vi "PH_ForceSensor.read DB.vi"(1 "Force Sensor Instance":string, 5 "error in (no error)":errorcluster) -> (13 "Ranges [N]":T1, 15 "Supply Voltage [V]":dbl, 16 "Full Force [N]":dbl, 17 "Offsets [µV]":T2, 18 "Scalings [mV/V]":T2, 19 "error out":errorcluster)   [LabVIEW 2014, in "PH_ForceSensor.lvlib"]
uses:
  PH_ForceSensor.lvlib
  PH_ForceSensor.Dataset.ctl
  PH_ForceSensor.Ranges.ctl
  PH_Common/PH_Common.lvlib
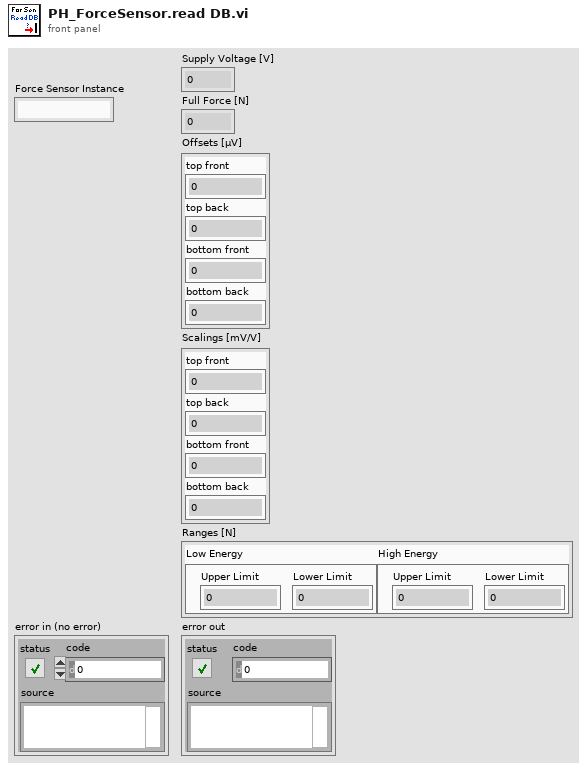
[diagram p1: front panel]
types:
  T1 = typedef "PH_ForceSensor.lvlib/PH_ForceSensor.Ranges.ctl" = cluster{"Low Energy":cluster{"Upper Limit":dbl, "Lower Limit":dbl}, "High Energy":cluster{"Upper Limit":dbl, "Lower Limit":dbl}}
  T2 = typedef "PH_ForceSensor.lvlib/PH_ForceSensor.Dataset.ctl" = cluster{"top front":dbl, "top back":dbl, "bottom front":dbl, "bottom back":dbl}
  T3 = cluster{"[0]":dbl, "[1]":dbl, "[2]":dbl, "[3]":dbl}
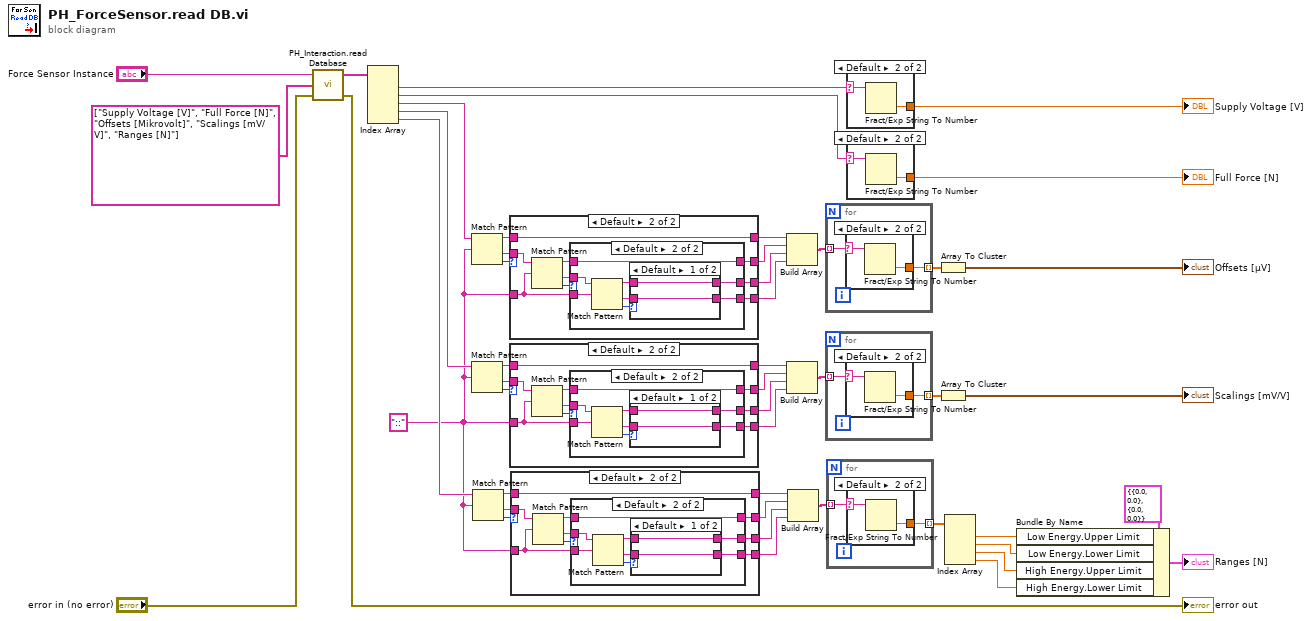
[diagram p0: block diagram]
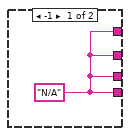
[diagram p2: hidden frame]
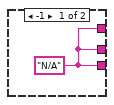
[diagram p3: hidden frame]
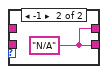
[diagram p4: hidden frame]
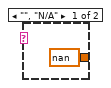
[diagram p5: hidden frame]
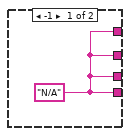
[diagram p6: hidden frame]
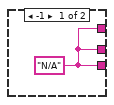
[diagram p7: hidden frame]
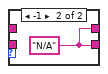
[diagram p8: hidden frame]
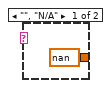
[diagram p9: hidden frame]
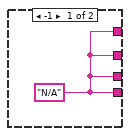
[diagram p10: hidden frame]
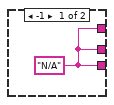
[diagram p11: hidden frame]
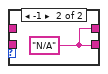
[diagram p12: hidden frame]
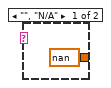
[diagram p13: hidden frame]
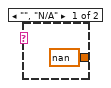
[diagram p14: hidden frame]
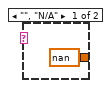
[diagram p15: hidden frame]
diagram:
  w1 = "::" ("regular expression")
  n1 = call "PH_Interaction.read Database.vi"("error in (no error)"="error in (no error)", "Strings to search for"=string[] ["Supply Voltage [V]", "Full Force [N]", "Offsets [Mikrovolt]", "Scalings [mV/V]", "Ranges [N]"], "DB Entry to read"="Force Sensor Instance") -> ("error out"=→"error out":errorcluster, "Values"=w48:string[])  [unwired: 1 in]
  n2 = Index Array(array=w48) -> (element #1=w42:string, element #2=w41:string, element #3=w39:string, element #4=w18:string, element #5=w9:string)  [unwired: 5 in]
  n3 = Match Pattern(string=w39, regular expression=w1) -> (before substring=w33:string, after substring=w38:string, offset past match=w31:i32)  [unwired: 1 in, 1 out]
  n4 = Match Pattern(string=w18, regular expression=w1) -> (before substring=w23:string, after substring=w28:string, offset past match=w21:i32)  [unwired: 1 in, 1 out]
  n5 = Match Pattern(string=w9, regular expression=w1) -> (before substring=w12:string, after substring=w17:string, offset past match=w10:i32)  [unwired: 1 in, 1 out]
  n6 = case shown="Default" w31 {
    tunnel: w38 -> [_ w58]
    tunnel: w1 -> [_ w56]
    tunnel: [w49 w55] -> w36
    tunnel: [w49 w54] -> w35
    tunnel: [w49 w51] -> w34
    tunnel: w33 -> [_ w50]
    tunnel: [w49 w50] -> w32
    frame -1 {
      w49 = "N/A"
    }
    frame Default {
      n7 = Match Pattern(string=w58, regular expression=w56) -> (before substring=w52:string, after substring=w57:string, offset past match=w53:i32)  [unwired: 1 in, 1 out]
      n8 = case shown="Default" w53 {
        tunnel: w57 -> [_ w67]
        tunnel: w56 -> [_ w66]
        tunnel: [w59 w64] -> w55
        tunnel: [w59 w61] -> w54
        tunnel: w52 -> [_ w60]
        tunnel: [w59 w60] -> w51
        frame -1 {
          w59 = "N/A"
        }
        frame Default {
          n9 = Match Pattern(string=w67, regular expression=w66) -> (before substring=w63:string, after substring=w62:string, offset past match=w65:i32)  [unwired: 1 in, 1 out]
          n10 = case shown="Default" w65 {
            tunnel: [w69 w70] -> w64
            tunnel: w63 -> [w69 _]
            tunnel: w62 -> [w68 _]
            tunnel: [w68 w70] -> w61
            frame Default {
            }
            frame -1 {
              w70 = "N/A"
            }
          }
        }
      }
    }
  }
  n11 = case shown="Default" w21 {
    tunnel: w28 -> [_ w80]
    tunnel: w1 -> [_ w78]
    tunnel: [w71 w77] -> w26
    tunnel: [w71 w76] -> w25
    tunnel: [w71 w73] -> w24
    tunnel: w23 -> [_ w72]
    tunnel: [w71 w72] -> w22
    frame -1 {
      w71 = "N/A"
    }
    frame Default {
      n12 = Match Pattern(string=w80, regular expression=w78) -> (before substring=w74:string, after substring=w79:string, offset past match=w75:i32)  [unwired: 1 in, 1 out]
      n13 = case shown="Default" w75 {
        tunnel: w79 -> [_ w89]
        tunnel: w78 -> [_ w88]
        tunnel: [w81 w86] -> w77
        tunnel: [w81 w83] -> w76
        tunnel: w74 -> [_ w82]
        tunnel: [w81 w82] -> w73
        frame -1 {
          w81 = "N/A"
        }
        frame Default {
          n14 = Match Pattern(string=w89, regular expression=w88) -> (before substring=w85:string, after substring=w84:string, offset past match=w87:i32)  [unwired: 1 in, 1 out]
          n15 = case shown="Default" w87 {
            tunnel: [w91 w92] -> w86
            tunnel: w85 -> [w91 _]
            tunnel: w84 -> [w90 _]
            tunnel: [w90 w92] -> w83
            frame Default {
            }
            frame -1 {
              w92 = "N/A"
            }
          }
        }
      }
    }
  }
  n16 = case shown="Default" w10 {
    tunnel: w17 -> [_ w102]
    tunnel: w1 -> [_ w100]
    tunnel: [w93 w99] -> w15
    tunnel: [w93 w98] -> w14
    tunnel: [w93 w95] -> w13
    tunnel: w12 -> [_ w94]
    tunnel: [w93 w94] -> w11
    frame -1 {
      w93 = "N/A"
    }
    frame Default {
      n17 = Match Pattern(string=w102, regular expression=w100) -> (before substring=w96:string, after substring=w101:string, offset past match=w97:i32)  [unwired: 1 in, 1 out]
      n18 = case shown="Default" w97 {
        tunnel: w101 -> [_ w111]
        tunnel: w100 -> [_ w110]
        tunnel: [w103 w108] -> w99
        tunnel: [w103 w105] -> w98
        tunnel: w96 -> [_ w104]
        tunnel: [w103 w104] -> w95
        frame -1 {
          w103 = "N/A"
        }
        frame Default {
          n19 = Match Pattern(string=w111, regular expression=w110) -> (before substring=w107:string, after substring=w106:string, offset past match=w109:i32)  [unwired: 1 in, 1 out]
          n20 = case shown="Default" w109 {
            tunnel: [w113 w114] -> w108
            tunnel: w107 -> [w113 _]
            tunnel: w106 -> [w112 _]
            tunnel: [w112 w114] -> w105
            frame Default {
            }
            frame -1 {
              w114 = "N/A"
            }
          }
        }
      }
    }
  }
  n21 = Build Array(w32, w34, w36, w35) -> (w37:string[])
  n22 = Build Array(w22, w24, w26, w25) -> (w27:string[])
  n23 = Build Array(w11, w13, w15, w14) -> (w16:string[])
  n24 = for {
    tunnel: w37 -> [w116] mode=indexing
    tunnel: [w115] -> w30 mode=indexing
    n25 = case shown="Default" w116 {
      selector: w116 -> [_ w118]
      tunnel: [nan w119] -> w115
      frame "", "N/A" {
      }
      frame Default {
        n26 = Fract/Exp String To Number(string=w118) -> (number=w119:dbl)  [unwired: 3 in, 1 out]
      }
    }
  }
  n27 = for {
    tunnel: w27 -> [w121] mode=indexing
    tunnel: [w120] -> w20 mode=indexing
    n28 = case shown="Default" w121 {
      selector: w121 -> [_ w123]
      tunnel: [nan w124] -> w120
      frame "", "N/A" {
      }
      frame Default {
        n29 = Fract/Exp String To Number(string=w123) -> (number=w124:dbl)  [unwired: 3 in, 1 out]
      }
    }
  }
  n30 = for {
    tunnel: w16 -> [w126] mode=indexing
    tunnel: [w125] -> w6 mode=indexing
    n31 = case shown="Default" w126 {
      selector: w126 -> [_ w128]
      tunnel: [nan w129] -> w125
      frame "", "N/A" {
      }
      frame Default {
        n32 = Fract/Exp String To Number(string=w128) -> (number=w129:dbl)  [unwired: 3 in, 1 out]
      }
    }
  }
  n33 = case shown="Default" w42 {
    selector: w42 -> [_ w131]
    tunnel: [nan w132] -> w43
    frame "", "N/A" {
    }
    frame Default {
      n34 = Fract/Exp String To Number(string=w131) -> (number=w132:dbl)  [unwired: 3 in, 1 out]
    }
  }
  "Supply Voltage [V]" <- w43
  n35 = case shown="Default" w41 {
    selector: w41 -> [_ w134]
    tunnel: [nan w135] -> w40
    frame "", "N/A" {
    }
    frame Default {
      n36 = Fract/Exp String To Number(string=w134) -> (number=w135:dbl)  [unwired: 3 in, 1 out]
    }
  }
  "Full Force [N]" <- w40
  n37 = Array To Cluster(array=w30) -> (cluster=→"Offsets [µV]":T3)
  n38 = Array To Cluster(array=w20) -> (cluster=→"Scalings [mV/V]":T3)
  n39 = Index Array(array=w6) -> (element #1=w5:dbl, element #2=w4:dbl, element #3=w3:dbl, element #4=w2:dbl)  [unwired: 4 in]
  n40 = Bundle By Name(cluster=T1 {"Low Energy"={"Upper Limit"=0.0, "Lower Limit"=0.0}, "High Energy"={"Upper Limit"=0.0, "Lower Limit"=0.0}} ("Ranges [N]"), "Low Energy.Upper Limit"=w5, "Low Energy.Lower Limit"=w4, "High Energy.Upper Limit"=w3, "High Energy.Lower Limit"=w2) -> (→"Ranges [N]":T1)
